vi "Subpanel VI.vi"() -> ()   [LabVIEW 2020, in "MacroAssert Tests.lvlib"]
uses:
  MacroAssert Tests.lvlib
panel:
  out "Status":string
  in  "Set Random Numeric":bool
  in  "Do Something":bool
  out "Numeric":dbl
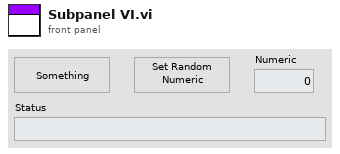
[diagram p1: front panel]
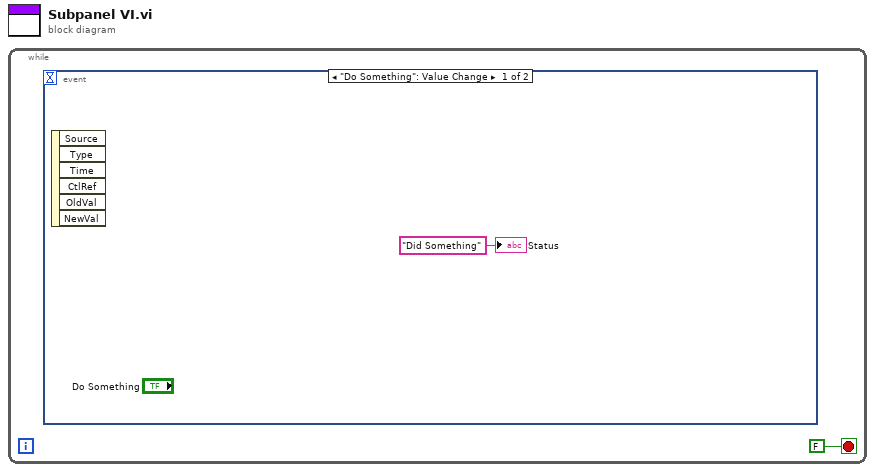
[diagram p0: block diagram]
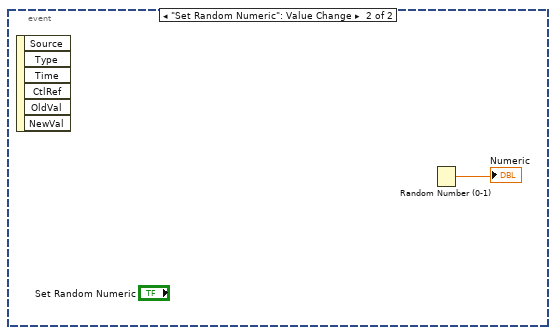
[diagram p2: hidden frame]
diagram:
  n1 = while {
    stop <- FALSE stop-if-true
    n2 = event shown="[0] \"Do Something\": Value Change" {
      selector: _ -> [_ _]
      dyn-events: _ -> [_ _]
      timeout: _ -> [_ _]
      event "Do Something": Value Change {
        n3 = event-data() -> ()  [unwired: 1 in, 6 out]
        "Status" <- "Did Something" ("Status")
      }
      event "Set Random Numeric": Value Change {
        n4 = event-data() -> ()  [unwired: 1 in, 6 out]
        n5 = Random Number (0-1)() -> (number: 0 to 1=→"Numeric":dbl)
      }
    }
  }
